vi "ReadCal.vi"() -> (0 "Informe":string, 1 "VelocitatMaxima":dbl caption="VelocitatMàxima", 2 "Deformacio":dbl, 3 "Velocitat":dbl, 4 "Taula":string[](array[string]), 5 "Password":string, 6 "Path":string)   [LabVIEW 2017]
uses:
  <vilib>/registry/registry.llb/Registry RtKey.ctl
  <vilib>/registry/registry.llb/Read Registry Value Simple STR.vi
panel:
  out "error out":errorcluster
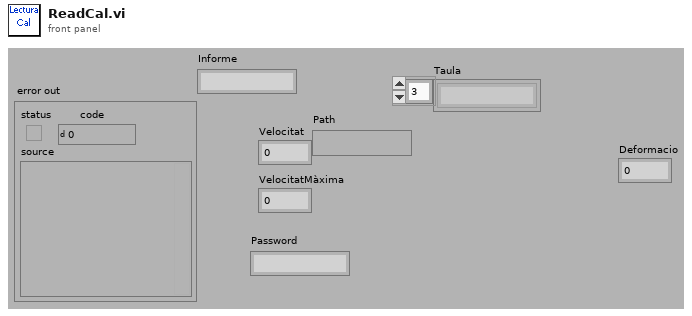
[diagram p1: front panel]
types:
  T1 = typedef "Registry RtKey.ctl" = enum32{"HKEY_CLASSES_ROOT", "HKEY_CURRENT_USER", "HKEY_LOCAL_MACHINE", "HKEY_USERS", "HKEY_PERFORMANCE_DATA", "HKEY_CURRENT_CONFIG", "HKEY_DYN_DATA"}
  T2 = typedef "Registry refnum.ctl" = refnum<k1>
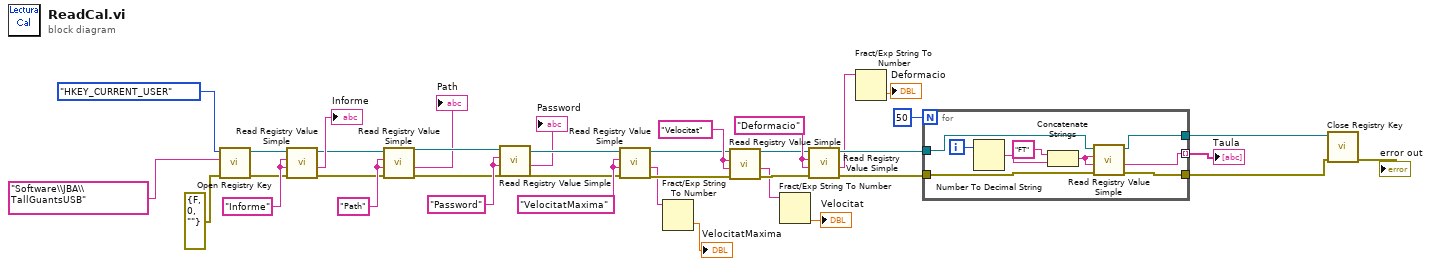
[diagram p0: block diagram]
diagram:
  w6 = "Path" ("value")
  w10 = "Informe" ("value")
  w12 = "Password" ("value")
  w19 = "VelocitatMaxima" ("value")
  w31 = "Velocitat" ("value")
  w33 = "Deformacio" ("value")
  n1 = call <vilib>:"Open Registry Key.vi"("error in (no error)"=errorcluster {"status"=FALSE, "code"=0, "source"=""}, "subkey"="Software\\JBA\\TallGuantsUSB", "root key (HKEY_LOCAL_MACHINE)"=Registry_RtKey."HKEY_CURRENT_USER") -> ("error out"=w8:errorcluster, "refnum out"=w9:T2)  [unwired: 7 in]
  n2 = call-poly <vilib>:"Read Registry Value Simple.vi"("error in (no error)"=w8, "default data"=w10, "value"=w10, "refnum"=w9) -> ("error out"=w4:errorcluster, "String/Binary data"=→"Informe":string, "refnum out"=w5:T2)  [unwired: 2 in, 1 out]
  n3 = call-poly <vilib>:"Read Registry Value Simple.vi"("error in (no error)"=w4, "default data"=w6, "value"=w6, "refnum"=w5) -> ("error out"=w3:errorcluster, "String/Binary data"=→"Path":string, "refnum out"=w2:T2)  [unwired: 2 in, 1 out]
  n4 = call-poly <vilib>:"Read Registry Value Simple.vi"("error in (no error)"=w3, "default data"=w12, "value"=w12, "refnum"=w2) -> ("error out"=w13:errorcluster, "String/Binary data"=→"Password":string, "refnum out"=w14:T2)  [unwired: 2 in, 1 out]
  n5 = call-poly <vilib>:"Read Registry Value Simple.vi"("error in (no error)"=w13, "default data"=w19, "value"=w19, "refnum"=w14) -> ("error out"=w17:errorcluster, "String/Binary data"=w16:string, "refnum out"=w18:T2)  [unwired: 2 in, 1 out]
  n6 = Fract/Exp String To Number(string=w16) -> (number=→"VelocitatMaxima":dbl)  [unwired: 3 in, 1 out]
  n7 = call-poly <vilib>:"Read Registry Value Simple.vi"("error in (no error)"=w17, "default data"=w31, "value"=w31, "refnum"=w18) -> ("error out"=w29:errorcluster, "String/Binary data"=w28:string, "refnum out"=w30:T2)  [unwired: 2 in, 1 out]
  n8 = Fract/Exp String To Number(string=w28) -> (number=→"Velocitat":dbl)  [unwired: 3 in, 1 out]
  n9 = call-poly <vilib>:"Read Registry Value Simple.vi"("error in (no error)"=w29, "default data"=w33, "value"=w33, "refnum"=w30) -> ("error out"=w35:errorcluster, "String/Binary data"=w32:string, "refnum out"=w34:T2)  [unwired: 2 in, 1 out]
  n10 = Fract/Exp String To Number(string=w32) -> (number=→"Deformacio":dbl)  [unwired: 3 in, 1 out]
  n11 = for {
    N: 50 -> [_]
    tunnel: w34 -> [w46]
    tunnel: w35 -> [w45]
    tunnel: [w41] -> w23
    tunnel: [w40] -> w24
    tunnel: [w38] -> w22 mode=indexing
    i -> [w44]
    n12 = Number To Decimal String(number=w44) -> (decimal integer string=w42:string)  [unwired: 1 in]
    n13 = Concatenate Strings("FT" ("value"), w42) -> (w39:string)
    n14 = call-poly <vilib>:"Read Registry Value Simple.vi"("error in (no error)"=w45, "default data"=w39, "value"=w39, "refnum"=w46) -> ("error out"=w41:errorcluster, "String/Binary data"=w38:string, "refnum out"=w40:T2)  [unwired: 2 in, 1 out]
  }
  "Taula" <- w22
  n15 = call <vilib>:"Close Registry Key.vi"("error in (no error)"=w23, "refnum"=w24) -> ("error out"=→"error out":errorcluster)  [unwired: 5 in]
